vi "test Enable Disable CD.vi"(8 "error in (no error)":errorcluster, 11 "TestCase in":refnum<class "Embedded Data Logger Scripting Unit Tests.lvclass">) -> (0 "error out":errorcluster, 3 "TestCase out":refnum<class "Embedded Data Logger Scripting Unit Tests.lvclass">)   [LabVIEW 2027, in "Embedded Data Logger Scripting Unit Tests.lvclass"]
uses:
  Embedded Data Logger Scripting Unit Tests.lvclass
  C:/Program Files/National Instruments/LabVIEW 2027/vi.lib/NI/VeriStand Custom Device Testing Tools/VeriStandScriptingTestCase/VeriStandScriptingTestCase.lvclass
  <vilib>/NI/VeriStand Custom Device Testing Tools/VeriStandScriptingTestCase/VeriStandScriptingTestCase.lvclass/VeriStandScriptingTestCase.ctl
  <vilib>/NI/VeriStand Custom Device Testing Tools/VeriStandScriptingTestCase/Read Target.vi
  C:/NetCoreDLL/NationalInstruments.VeriStand.SystemDefinitionAPI.dll
  NetCoreDLL/NationalInstruments.VeriStand.SystemDefinitionAPI.dll
  C:/Program Files/National Instruments/LabVIEW 2027/vi.lib/addons/_JKI Toolkits/VI Tester/TestCase.llb/TestCase.lvclass
  <vilib>/addons/_JKI Toolkits/VI Tester/TestCase.llb/TestCase.lvclass
  Embedded Data Logger Scripting.lvlib
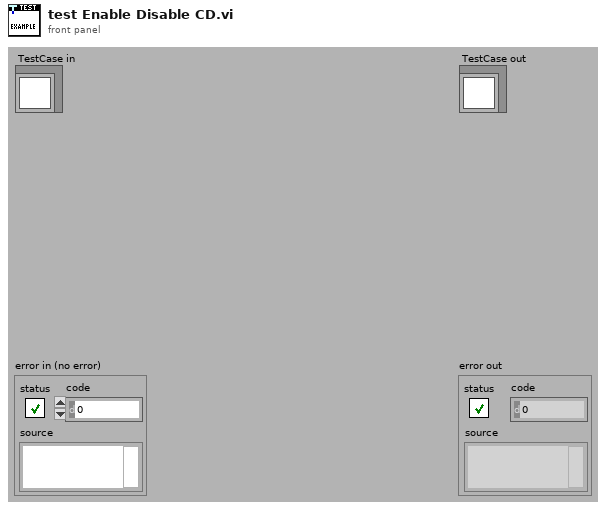
[diagram p1: front panel]
types:
  T1 = typedef "Custom Device API.lvlib/Custom Device Item Ref.ctl" = u64
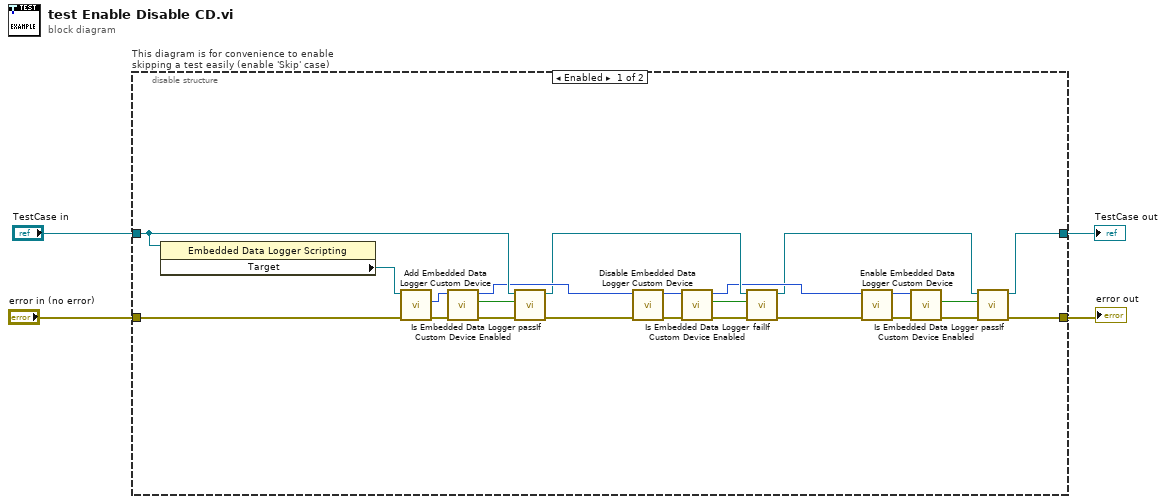
[diagram p0: block diagram]
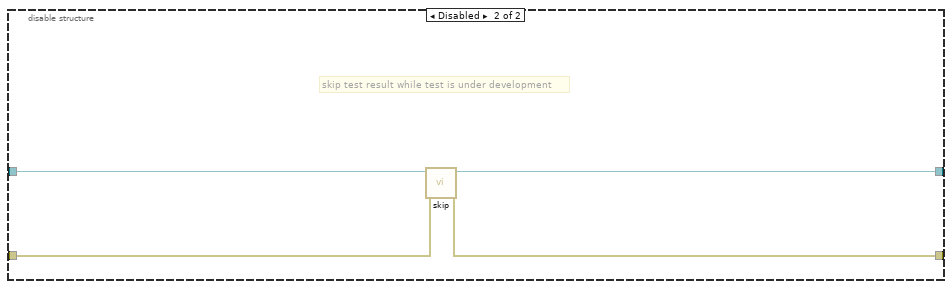
[diagram p2: hidden frame]
diagram:
  n1 = disable-structure "This diagram is for convenience to enable skipping a test easily (enable 'Skip' case)" shown="Enabled" {
    disable-tunnel: "TestCase in" -> [w21 w31]
    disable-tunnel: [w5 w29] -> w1
    disable-tunnel: [w7 w30] -> w3
    disable-tunnel: "error in (no error)" -> [w26 w28]
    frame Enabled {
      n2 = property class="Embedded Data Logger Scripting "(reference=w21) -> ("Target"=w27:refnum<k39>)  [unwired: 1 in, 2 out]
      n3 = call "Add Embedded Data Logger Custom Device.vi"("error in"=w26, "NationalInstruments.VeriStand.SystemDefinitionAPI.Target"=w27) -> ("error out"=w25:errorcluster, "embedded data logger"=w24:T1)  [unwired: 7 in, 1 out]
      n4 = call "Is Embedded Data Logger Custom Device Enabled.vi"("error in"=w25, "embedded data logger in"=w24) -> ("error out"=w23:errorcluster, "enabled"=w22:bool, "embedded data logger out"=w19:T1)  [unwired: 7 in]
      n5 = call-dynamic "passIf.vi"("error in (no error)"=w23, "pass"=w22, "TestCase in"=w21) -> ("error out"=w20:errorcluster, "TestCase out"=w14:refnum<class "Embedded Data Logger Scripting Unit Tests.lvclass">)  [unwired: 7 in]
      n6 = call "Disable Embedded Data Logger Custom Device.vi"("error in"=w20, "embedded data logger in"=w19) -> ("error out"=w18:errorcluster, "embedded data logger out"=w17:T1)  [unwired: 8 in]
      n7 = call "Is Embedded Data Logger Custom Device Enabled.vi"("error in"=w18, "embedded data logger in"=w17) -> ("error out"=w16:errorcluster, "enabled"=w15:bool, "embedded data logger out"=w12:T1)  [unwired: 7 in]
      n8 = call-dynamic "failIf.vi"("error in (no error)"=w16, "fail"=w15, "TestCase in"=w14) -> ("error out"=w13:errorcluster, "TestCase out"=w6:refnum<class "Embedded Data Logger Scripting Unit Tests.lvclass">)  [unwired: 7 in]
      n9 = call "Enable Embedded Data Logger Custom Device.vi"("error in"=w13, "embedded data logger in"=w12) -> ("error out"=w8:errorcluster, "embedded data logger out"=w9:T1)  [unwired: 8 in]
      n10 = call "Is Embedded Data Logger Custom Device Enabled.vi"("error in"=w8, "embedded data logger in"=w9) -> ("error out"=w10:errorcluster, "enabled"=w11:bool)  [unwired: 7 in, 1 out]
      n11 = call-dynamic "passIf.vi"("error in (no error)"=w10, "pass"=w11, "TestCase in"=w6) -> ("error out"=w7:errorcluster, "TestCase out"=w5:refnum<class "Embedded Data Logger Scripting Unit Tests.lvclass">)  [unwired: 7 in]
    }
    frame Disabled {
      # "skip test result while test is under development"
      n12 = call <vilib>:"skip.vi"("error in (no error)"=w28, "TestCase in"=w31) -> ("error out"=w30:errorcluster, "TestCase out"=w29:refnum<class "Embedded Data Logger Scripting Unit Tests.lvclass">)  [unwired: 8 in]
    }
  }
  "error out" <- w3
  "TestCase out" <- w1
